vi "RichToFlatnidaqmx_grpc_GetChanAttributeStringRequest.vi"(5 "OutputClusterType":T1, 11 "InputCluster":T4) -> (3 "OutputCluster":T1)   [LabVIEW 2021, in "NI_DAQmx_client.lvlib"]
uses:
  NI_DAQmx_client.lvlib
  nidaqmx_grpc_GetChanAttributeStringRequest.ctl
  nidevice_grpc_Session_session/nidevice_grpc_Session_session.lvclass
  nidaqmx_grpc_GetChanAttributeStringRequest_attribute_enum/nidaqmx_grpc_GetChanAttributeStringRequest_attribute_enum.lvclass
  nidevice_grpc_Session.ctl
  nidaqmx_grpc_GetChanAttributeStringRequest_Flat.ctl
  nidevice_grpc_Session_Flat.ctl
  nidaqmx_grpc_ChannelStringAttribute.ctl
  nidevice_grpc_Session_session/nidevice_grpc_Session_session.lvclass/nidevice_grpc_Session_session.ctl
  nidaqmx_grpc_GetChanAttributeStringRequest_attribute_enum/nidaqmx_grpc_GetChanAttributeStringRequest_attribute_enum.lvclass/nidaqmx_grpc_GetChanAttributeStringRequest_attribute_enum.ctl
  nidevice_grpc_Session_session/Getname.vi
  nidevice_grpc_Session_session/Getid.vi
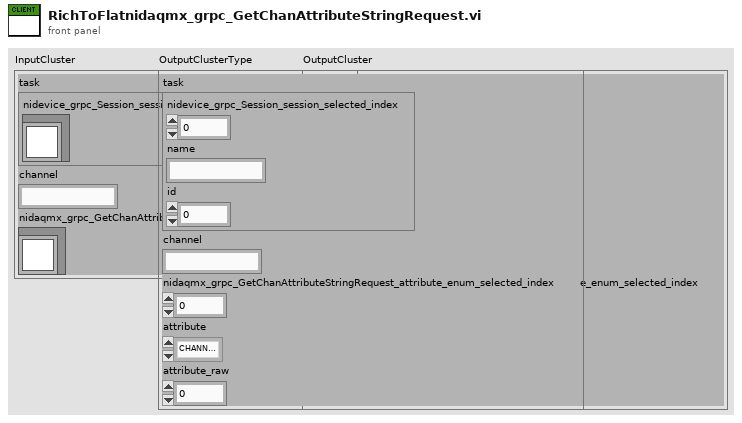
[diagram p1: front panel]
types:
  T1 = typedef "NI_DAQmx_client.lvlib/nidaqmx_grpc_GetChanAttributeStringRequest_Flat.ctl" = cluster{"task":T2, "channel":string, "nidaqmx_grpc_GetChanAttributeStringRequest_attribute_enum_selected_index":i32, "attribute":T3, "attribute_raw":i32}
  T2 = typedef "NI_DAQmx_client.lvlib/nidevice_grpc_Session_Flat.ctl" = cluster{"nidevice_grpc_Session_session_selected_index":i32, "name":string, "id":u32}
  T3 = typedef "NI_DAQmx_client.lvlib/nidaqmx_grpc_ChannelStringAttribute.ctl" = enum32{"CHANNEL_STRING_ATTRIBUTE_UNSPECIFIED", "CHANNEL_ATTRIBUTE_CI_CTR_TIMEBASE_SRC", "CHANNEL_ATTRIBUTE_CO_CTR_TIMEBASE_SRC", "CHANNEL_ATTRIBUTE_AI_THRMCPL_CJC_CHAN", "CHANNEL_ATTRIBUTE_CI_GPS_SYNC_SRC", "CHANNEL_ATTRIBUTE_AO_CUSTOM_SCALE_NAME", "CHANNEL_ATTRIBUTE_AI_CUSTOM_SCALE_NAME", "CHANNEL_ATTRIBUTE_CI_CUSTOM_SCALE_NAME", "CHANNEL_ATTRIBUTE_CI_FREQ_TERM", "CHANNEL_ATTRIBUTE_CI_PERIOD_TERM", "CHANNEL_ATTRIBUTE_CI_PULSE_WIDTH_TERM", "CHANNEL_ATTRIBUTE_CI_TWO_EDGE_SEP_FIRST_TERM", "CHANNEL_ATTRIBUTE_CI_TWO_EDGE_SEP_SECOND_TERM", "CHANNEL_ATTRIBUTE_CI_SEMI_PERIOD_TERM", "CHANNEL_ATTRIBUTE_CI_COUNT_EDGES_TERM", "CHANNEL_ATTRIBUTE_CO_PULSE_TERM", "CHANNEL_ATTRIBUTE_PHYSICAL_CHAN_NAME", "CHANNEL_ATTRIBUTE_CHAN_DESCR", "CHANNEL_ATTRIBUTE_AI_INPUT_SRC", "CHANNEL_ATTRIBUTE_CI_ENCODER_A_INPUT_TERM", "CHANNEL_ATTRIBUTE_CI_ENCODER_B_INPUT_TERM", "CHANNEL_ATTRIBUTE_CI_ENCODER_Z_INPUT_TERM", "CHANNEL_ATTRIBUTE_AI_TEDS_UNITS", "CHANNEL_ATTRIBUTE_CI_COUNT_EDGES_DIR_TERM", "CHANNEL_ATTRIBUTE_CI_FREQ_DIG_FLTR_TIMEBASE_SRC", "CHANNEL_ATTRIBUTE_CI_PERIOD_DIG_FLTR_TIMEBASE_SRC", "CHANNEL_ATTRIBUTE_CI_COUNT_EDGES_COUNT_DIR_DIG_FLTR_TIMEBASE_SRC", "CHANNEL_ATTRIBUTE_CI_COUNT_EDGES_DIG_FLTR_TIMEBASE_SRC", "CHANNEL_ATTRIBUTE_CI_ENCODER_A_INPUT_DIG_FLTR_TIMEBASE_SRC", "CHANNEL_ATTRIBUTE_CI_ENCODER_B_INPUT_DIG_FLTR_TIMEBASE_SRC", "CHANNEL_ATTRIBUTE_CI_ENCODER_Z_INPUT_DIG_FLTR_TIMEBASE_SRC", "CHANNEL_ATTRIBUTE_CI_PULSE_WIDTH_DIG_FLTR_TIMEBASE_SRC", "CHANNEL_ATTRIBUTE_CI_TWO_EDGE_SEP_FIRST_DIG_FLTR_TIMEBASE_SRC", "CHANNEL_ATTRIBUTE_CI_TWO_EDGE_SEP_SECOND_DIG_FLTR_TIMEBASE_SRC", "CHANNEL_ATTRIBUTE_CI_SEMI_PERIOD_DIG_FLTR_TIMEBASE_SRC", "CHANNEL_ATTRIBUTE_AO_DAC_REF_EXT_SRC", "CHANNEL_ATTRIBUTE_AO_DAC_OFFSET_EXT_SRC", "CHANNEL_ATTRIBUTE_CI_CTR_TIMEBASE_DIG_FLTR_TIMEBASE_SRC", "CHANNEL_ATTRIBUTE_CO_CTR_TIMEBASE_DIG_FLTR_TIMEBASE_SRC", "CHANNEL_ATTRIBUTE_AI_CHAN_CAL_OPERATOR_NAME", "CHANNEL_ATTRIBUTE_AI_CHAN_CAL_DESC", "CHANNEL_ATTRIBUTE_DI_DIG_FLTR_TIMEBASE_SRC", "CHANNEL_ATTRIBUTE_CI_PULSE_FREQ_TERM", "CHANNEL_ATTRIBUTE_CI_PULSE_FREQ_DIG_FLTR_TIMEBASE_SRC", "CHANNEL_ATTRIBUTE_CI_PULSE_TIME_TERM", "CHANNEL_ATTRIBUTE_CI_PULSE_TIME_DIG_FLTR_TIMEBASE_SRC", "CHANNEL_ATTRIBUTE_CI_PULSE_TICKS_TERM", "CHANNEL_ATTRIBUTE_CI_PULSE_TICKS_DIG_FLTR_TIMEBASE_SRC", "CHANNEL_ATTRIBUTE_CI_COUNT_EDGES_COUNT_RESET_TERM", "CHANNEL_ATTRIBUTE_CI_COUNT_EDGES_COUNT_RESET_DIG_FLTR_TIMEBASE_SRC", "CHANNEL_ATTRIBUTE_AI_ROSETTE_STRAIN_GAGE_STRAIN_CHANS", "CHANNEL_ATTRIBUTE_CI_TIMESTAMP_TERM", "CHANNEL_ATTRIBUTE_NAV_CUSTOM_SCALE_NAME", "CHANNEL_ATTRIBUTE_CI_DUTY_CYCLE_TERM", "CHANNEL_ATTRIBUTE_CI_DUTY_CYCLE_DIG_FLTR_TIMEBASE_SRC", "CHANNEL_ATTRIBUTE_CI_VELOCITY_ENCODER_A_INPUT_TERM", "CHANNEL_ATTRIBUTE_CI_VELOCITY_ENCODER_A_INPUT_DIG_FLTR_TIMEBASE_SRC", "CHANNEL_ATTRIBUTE_CI_VELOCITY_ENCODER_B_INPUT_TERM", "CHANNEL_ATTRIBUTE_CI_VELOCITY_ENCODER_B_INPUT_DIG_FLTR_TIMEBASE_SRC", "CHANNEL_ATTRIBUTE_CI_COUNT_EDGES_GATE_TERM", "CHANNEL_ATTRIBUTE_CI_COUNT_EDGES_GATE_DIG_FLTR_TIMEBASE_SRC"}
  T4 = typedef "NI_DAQmx_client.lvlib/nidaqmx_grpc_GetChanAttributeStringRequest.ctl" = cluster{"task":T5, "channel":string, "nidaqmx_grpc_GetChanAttributeStringRequest_attribute_enum":refnum<class "nidaqmx_grpc_GetChanAttributeStringRequest_attribute_enum.lvclass">}
  T5 = typedef "NI_DAQmx_client.lvlib/nidevice_grpc_Session.ctl" = cluster{"nidevice_grpc_Session_session":refnum<class "nidevice_grpc_Session_session.lvclass">}
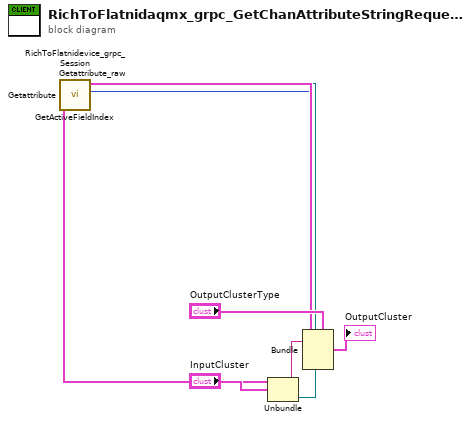
[diagram p0: block diagram]
diagram:
  n1 = Unbundle "Unbundle"("InputCluster") -> ("task"=w7:T5, "channel"=w5:string, "nidaqmx_grpc_GetChanAttributeStringRequest_attribute_enum"=w4:refnum<class "nidaqmx_grpc_GetChanAttributeStringRequest_attribute_enum.lvclass">)
  n2 = call "Getattribute_raw.vi"("OneOfTemplate in"=w4) -> ("Get_Val"=w1:i32)  [unwired: 8 in, 2 out]
  n3 = call "Getattribute.vi"("OneOfTemplate in"=w4) -> ("Get_Val"=w2:T3)  [unwired: 8 in, 2 out]
  n4 = call "GetActiveFieldIndex.vi"("OneOfTemplate in"=w4) -> ("Active Field Index"=w3:i32)  [unwired: 8 in, 2 out]
  n5 = call "RichToFlatnidevice_grpc_Session.vi"("InputCluster"=w7) -> ("OutputCluster"=w6:T2)  [unwired: 10 in]
  n6 = Bundle "Bundle"(cluster="OutputClusterType", "task"=w6, "channel"=w5, "nidaqmx_grpc_GetChanAttributeStringRequest_attribute_enum_selected_index"=w3, "attribute"=w2, "attribute_raw"=w1) -> (→"OutputCluster":T1)
